vi "Subvi detector change U16.vi"(9 "Input":u16) -> (1 "Output":bool)   [LabVIEW 2017]
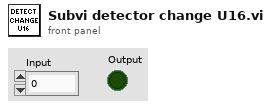
[diagram p1: front panel]
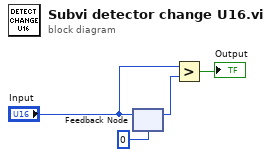
[diagram p0: block diagram]
diagram:
  n1 = feedback-in #1("Input") -> ()
  n2 = feedback #1(u16 0) -> (w3:u16)
  n3 = Greater?(x="Input", y=w3) -> (0:→"Output":bool)
